vi "getFlags.vi"(11 "PUBLISH in":refnum<class "PUBLISH.lvclass">) -> (0 "RETAIN":bool, 1 "QoS":T1, 2 "DUP":bool, 3 "PUBLISH out":refnum<class "PUBLISH.lvclass">)   [LabVIEW 2013, in "MQTT_Control_Packets.lvlib" / "PUBLISH.lvclass"]
uses:
  PUBLISH.lvclass
  ControlPacket/QualityOfService -- enum.ctl
  ControlPacket/ControlPacket.lvclass/ControlPacket.ctl
  ControlPacket/ControlPacket.lvclass
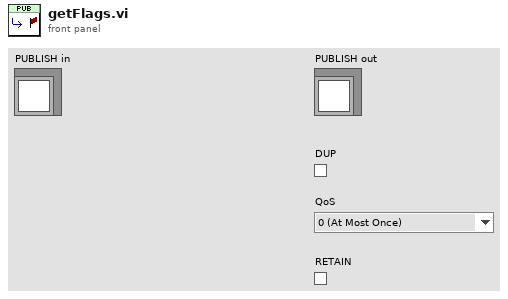
[diagram p1: front panel]
types:
  T1 = typedef "MQTT_Control_Packets.lvlib/ControlPacket.lvclass/QualityOfService -- enum.ctl" = enum16{"0 (At Most Once)", "1 (At Least Once)", "2 (Exactly Once)"}
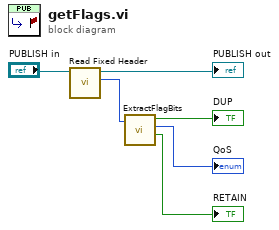
[diagram p0: block diagram]
diagram:
  n1 = call "Read Fixed Header.vi"("ControlPacket in"="PUBLISH in") -> ("Fixed Header"=w5:u8, "ControlPacket out"=→"PUBLISH out":refnum<class "PUBLISH.lvclass">)  [unwired: 9 in]
  n2 = call "ExtractFlagBits.vi"("Fixed Header"=w5) -> ("RETAIN"=→"RETAIN":bool, "QoS"=→"QoS":T1, "DUP"=→"DUP":bool)  [unwired: 7 in, 1 out]
